vi "Score_Elevators.vi"(0 "Hall Up/Down":T2, 1 "Elevator Up/Down":T2, 2 "Desired Floor":i32, 3 "Current Floor":i32, 4 "Car Calls for Each Floor":T1=[FALSE, FALSE, FALSE, FALSE], 5 "error in (no error)":errorcluster) -> (15 "Score":i32, 19 "error out":errorcluster)   [LabVIEW 2026]
uses:
  Controls/Motion_Status_Enum.ctl
  Controls/Car_Calls_Status.ctl
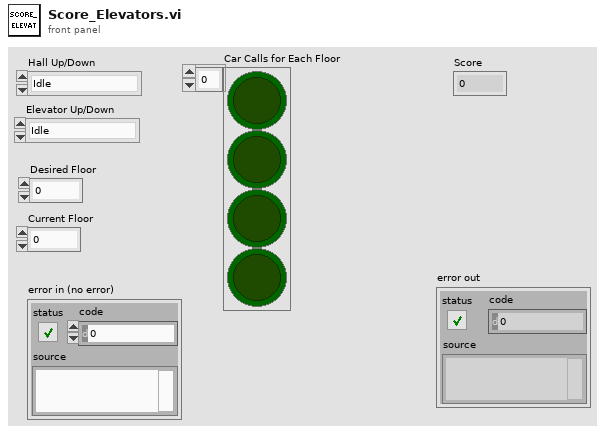
[diagram p1: front panel]
types:
  T1 = typedef "Car_Calls_Status.ctl" = bool[]
  T2 = typedef "Motion_Status_Enum.ctl" = enum16{"Idle", "Up", "Down"}
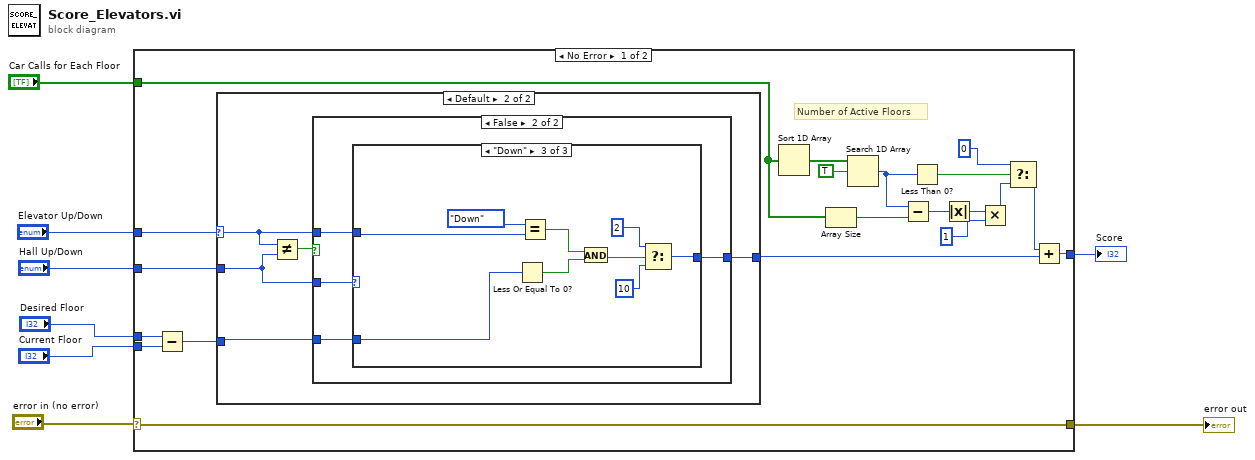
[diagram p0: block diagram]
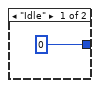
[diagram p2: hidden frame]
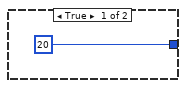
[diagram p3: hidden frame]
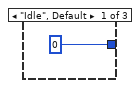
[diagram p4: hidden frame]
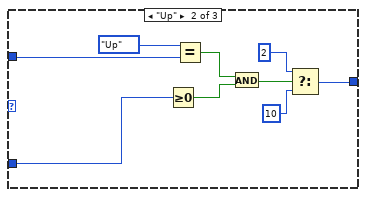
[diagram p5: hidden frame]
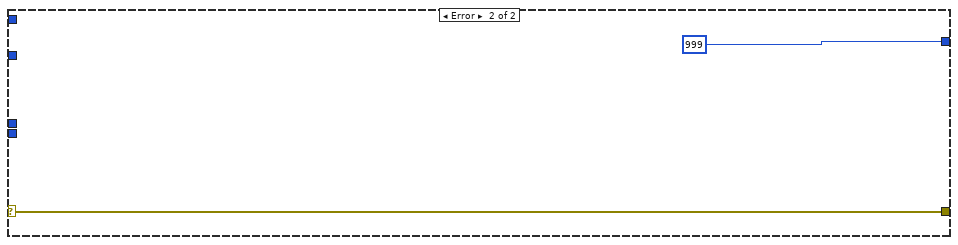
[diagram p6: hidden frame]
diagram:
  n1 = case shown="No Error" "error in (no error)" {
    selector: "error in (no error)" -> [w23 w59]
    tunnel: "Desired Floor" -> [w28 _]
    tunnel: "Current Floor" -> [w27 _]
    tunnel: "Hall Up/Down" -> [w25 _]
    tunnel: "Elevator Up/Down" -> [w24 _]
    tunnel: [w18 999 ("t")] -> w4
    tunnel: [w23 w59] -> w2
    tunnel: "Car Calls for Each Floor" -> [w19 _]
    frame No Error {
      # "Number of Active Floors"
      n2 = Subtract(x=w28, y=w27) -> (x-y=w26:i32)
      n3 = case shown="Default" w24 {
        selector: w24 -> [_ w30]
        tunnel: w25 -> [_ w32]
        tunnel: w26 -> [_ w31]
        tunnel: [0 w33] -> w17
        frame "Idle" {
        }
        frame Default {
          n4 = Not Equal?(x=w30, y=w32) -> (x != y?=w34:bool)
          n5 = case shown="False" w34 {
            tunnel: [20 w37] -> w33
            tunnel: w32 -> [_ w39]
            tunnel: w31 -> [_ w38]
            tunnel: w30 -> [_ w36]
            frame True {
            }
            frame False {
              n6 = case shown="\"Down\"" w39 {
                tunnel: [0 ("t") w43 w52] -> w37
                tunnel: w38 -> [_ w42 w51]
                tunnel: w36 -> [_ w41 w50]
                frame "Idle", Default {
                }
                frame "Up" {
                  n7 = Greater Or Equal To 0?(x=w42) -> (x >= 0?=w47:bool)
                  n8 = Equal?(x=Motion_Status_Enum."Up" ("value"), y=w41) -> (x = y?=w48:bool)
                  n9 = And(x=w48, y=w47) -> (x .and. y?=w44:bool)
                  n10 = Select(t=2, s=w44, f=10 ("t")) -> (s? t:f=w43:i32)
                }
                frame "Down" {
                  n11 = Less Or Equal To 0?(x=w51) -> (x <= 0?=w56:bool)
                  n12 = Equal?(x=Motion_Status_Enum."Down" ("value"), y=w50) -> (x = y?=w57:bool)
                  n13 = And(x=w57, y=w56) -> (x .and. y?=w53:bool)
                  n14 = Select(t=2, s=w53, f=10 ("t")) -> (s? t:f=w52:i32)
                }
              }
            }
          }
        }
      }
      n15 = Sort 1D Array(array=w19) -> (sorted array=w16:T1)
      n16 = Array Size(array=w19) -> (size(s)=w21:i32)
      n17 = Search 1D Array(1D array=w16, element=TRUE) -> (index of element=w13:i32)  [unwired: 1 in]
      n18 = Subtract(x=w13, y=w21) -> (x-y=w12:i32)
      n19 = Less Than 0?(x=w13) -> (x < 0?=w14:bool)
      n20 = Absolute Value(x=w12) -> (abs(x)=w11:i32)
      n21 = Multiply(x=w11, y=1) -> (x*y=w10:i32)
      n22 = Select(t=0 ("y"), s=w14, f=w10) -> (s? t:f=w9:i32)
      n23 = Add(x=w9, y=w17) -> (x+y=w18:i32)
    }
    frame Error {
    }
  }
  "Score" <- w4
  "error out" <- w2
